vi "PH_Revolver-GUI_6P.PC Write PSDB.vi"(0 "i ref in":refnum<vi>, 5 "error IO":errorcluster) -> (14 "i ref out":refnum<vi>, 19 "error out":errorcluster)   [LabVIEW 2014, in "PH_Revolver-GUI_6P.lvlib"]
doc: "This is the proc case which writes data to the PHELIX shot data base."
uses:
  PH_Revolver-GUI_6P.lvlib
  PH_4_Pos_Selector/PH_4_Pos_Selector.Position Selector.ctl
  PH_PSDBWriter/PH_PSDBWriter.lvlib
  PH_4_Pos_Selector/PH_4_Pos_Selector.lvlib
panel:
  in  "Current Position":T1 items=["unknown", "Position I", "Position II", "Position III", "Position IV", "moving"]
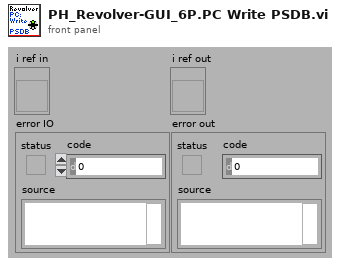
[diagram p1: front panel]
types:
  T1 = typedef "PH_4_Pos_Selector.lvlib/PH_4_Pos_Selector.Position Selector.ctl" = u16
  T2 = typedef "PH_Revolver-GUI_6P.lvlib/PH_Revolver-GUI_6P.i attribute.ctl" = cluster{"GUI Refs":cluster{"0°":refnum<vi>, "60°":refnum<vi>, "120°":refnum<vi>, "180°":refnum<vi>, "240°":refnum<vi>, "300°":refnum<vi>, "Action":refnum<vi>}, "Revolver Position":T3, "Service ID Position":i32, "Captions":string[]}
  T3 = typedef "PH_Revolver-GUI_6P.lvlib/PH_Revolver-GUI_6P.Position.ctl" = u16
  T4 = typedef "PH_PSDBWriter.lvlib/PH_PSDBWriter.String dataset.ctl" = cluster{"name":string, "data":string, "unit":string}
  T5 = typedef "PH_PSDBWriter.lvlib/PH_PSDBWriter.PSDB Dataset.ctl" = cluster{"Version":i32, "2D data Input":T6[], "Boolean Input":T8[], "Image Input":T9[], "Numeric Input":T11[], "String Input":T4[]}
  T6 = typedef "PH_PSDBWriter.lvlib/PH_PSDBWriter.2D dataset.ctl" = cluster{"name":string, "data":dbl[][], "axis description":T7}
  T7 = typedef "PSDB.lvlib/PSDB_AxisDescription.ctl" = cluster{"x axis label":string, "y axis label":string, "x axis unit":string, "y axis unit":string}
  T8 = typedef "PH_PSDBWriter.lvlib/PH_PSDBWriter.Boolean dataset.ctl" = cluster{"name":string, "data":bool, "unit":string}
  T9 = typedef "PH_PSDBWriter.lvlib/PH_PSDBWriter.Image dataset.ctl" = cluster{"name":string, "data":T10, "unit":string}
  T10 = typedef "IMAQ Image.ctl" = refnum<image>
  T11 = typedef "PH_PSDBWriter.lvlib/PH_PSDBWriter.Numeric dataset.ctl" = cluster{"name":string, "data":dbl, "unit":string}
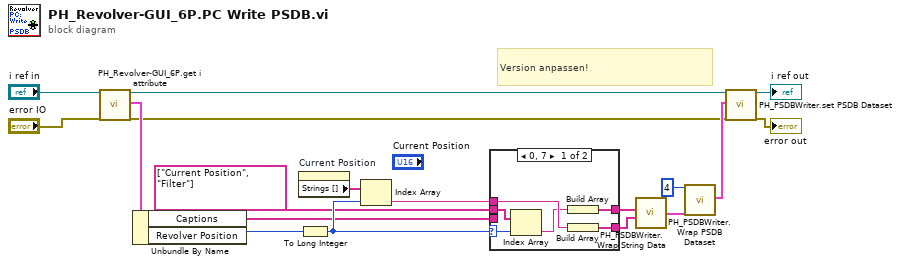
[diagram p0: block diagram]
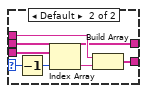
[diagram p2: hidden frame]
diagram:
  # "Version anpassen!"
  n1 = call "PH_Revolver-GUI_6P.get i attribute.vi"("i ref in"="i ref in", "error in (no error)"="error IO") -> ("i ref out"=w5:refnum<vi>, "i attribute"=w18:T2, "error out"=w4:errorcluster)  [unwired: 15 in]
  n2 = Unbundle By Name(w18) -> ("Captions"=w3:string[], "Revolver Position"=w16:T3)
  n3 = property on="Current Position" class="Ring (strict)"() -> ("Strings []"=w17:string[])  [unwired: 2 in, 2 out]
  n4 = To Long Integer(number=w16) -> (32bit integer=w14:i32)
  n5 = Index Array(array=w17, index=w14) -> (element=w15:string)
  n6 = case shown="0, 7" w14 {
    selector: w14 -> [w22 w26]
    tunnel: [w19 w25] -> w9
    tunnel: w15 -> [w24 w31]
    tunnel: [w23 w30] -> w10
    tunnel: w3 -> [_ w29]
    tunnel: string[] ["Current Position", "Filter"] -> [w21 w25]
    frame 0, 7 {
      n7 = Index Array(array=w21, index=w22) -> (element=w20:string)
      n8 = Build Array(w20) -> (w19:string[])
      n9 = Build Array(w24) -> (w23:string[])
    }
    frame Default {
      n10 = Decrement(x=w26) -> (x-1=w27:i32)
      n11 = Index Array(array=w29, index=w27) -> (element=w28:string)
      n12 = Build Array(w31, w28) -> (w30:string[])
    }
  }
  n13 = call "PH_PSDBWriter.Wrap String Data.vi"("Data Array"=w10, "Name Array"=w9) -> ("PSDB String Data Array"=w8:T4[])  [unwired: 2 in]
  n14 = call "PH_PSDBWriter.Wrap PSDB Dataset.vi"("Version"=4, "String Input"=w8) -> ("PSDB Dataset"=w7:T5)  [unwired: 17 in]
  n15 = call "PH_PSDBWriter.set PSDB Dataset.vi"("VI in"=w5, "PSDB Dataset"=w7, "error in (no error)"=w4) -> ("VI out"=→"i ref out":refnum<vi>, "error out"=→"error out":errorcluster)  [unwired: 15 in]
